vi "Get Favorite Color.vi"(8 "error in":errorcluster, 11 "DNatt in":refnum<class "DNatt.lvclass">) -> (0 "error out":errorcluster, 2 "Favorite Color":u32(colorbox), 3 "DNatt out":refnum<class "DNatt.lvclass">)   [LabVIEW 2024, in "DNatt.lvclass"]
uses:
  DNatt.lvclass
  DNatt.lvclass/DNatt.ctl
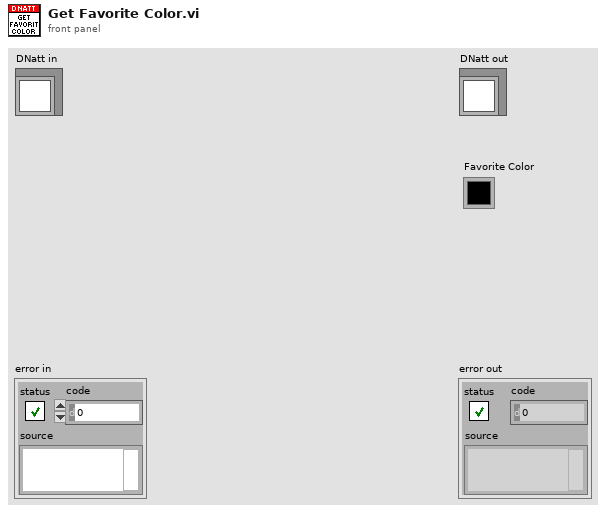
[diagram p1: front panel]
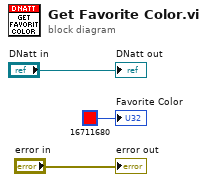
[diagram p0: block diagram]
diagram:
  "error out" <- "error in"
  "DNatt out" <- "DNatt in"
  "Favorite Color" <- u32 16711680
